vi "List Plugins.vi"(8 "error in (no error)":errorcluster, 11 "Parent Class":refnum<class "uPluggable.lvclass">) -> (0 "error out":errorcluster, 1 "Plugins' IDNs":string[](array[string]))   [LabVIEW 2021, in "uPlug.lvlib" / "uPlugin_Handler.lvclass"]
doc: "Pass in an interface class and get a list of all the IDN strings available as plugins for that interface."
uses:
  uPlugin_Handler.lvclass
  uPlugin_Handler.lvclass/uPlugin_Handler.ctl
  TypeDef_FGV Actions.ctl
  uPluggable/uPluggable.lvclass
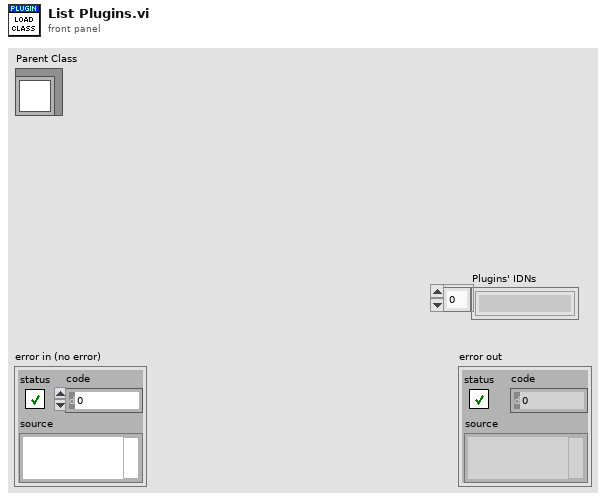
[diagram p1: front panel]
types:
  T1 = typedef "uPlug.lvlib/uPlugin_Handler.lvclass/TypeDef_FGV Actions.ctl" = enum16{"Init", "Load", "list"}
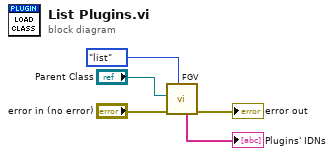
[diagram p0: block diagram]
diagram:
  n1 = call "FGV.vi"("Action"=TypeDef_FGV_Actions."list", "error in (no error)"="error in (no error)", "Parent Class"="Parent Class") -> ("error out"=→"error out":errorcluster, "Plugins' IDNs"=→"Plugins' IDNs":string[])  [unwired: 6 in, 1 out]
